vi "DataFlowExamples.vi"() -> ()   [LabVIEW 2020]
doc: "This VI have four examples of data flow using with good and bad habbits. Comments in polish language."
panel:
  out "Obecny czas 2":timestamp
  in  "Liczba 6":dbl
  in  "Liczba 5":dbl
  out "Wynik 3":dbl
  out "Obecny czas 1":timestamp
  out "Wynik 4":dbl
  in  "Liczba 7":dbl
  in  "Liczba 8":dbl
  in  "Liczba 3":dbl
  in  "Liczba 4":dbl
  out "Wynik 2":dbl
  out "Wynik 1":dbl
  in  "Liczba 2":dbl
  in  "Liczba 1":dbl
  # "Przykład 1"
  # "Przykład 2"
  # "Przykład 3"
  # "Przykład 4"
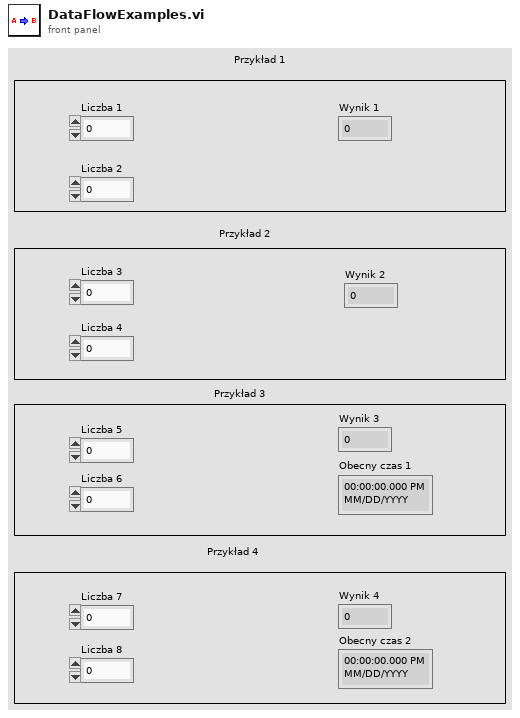
[diagram p1: front panel]
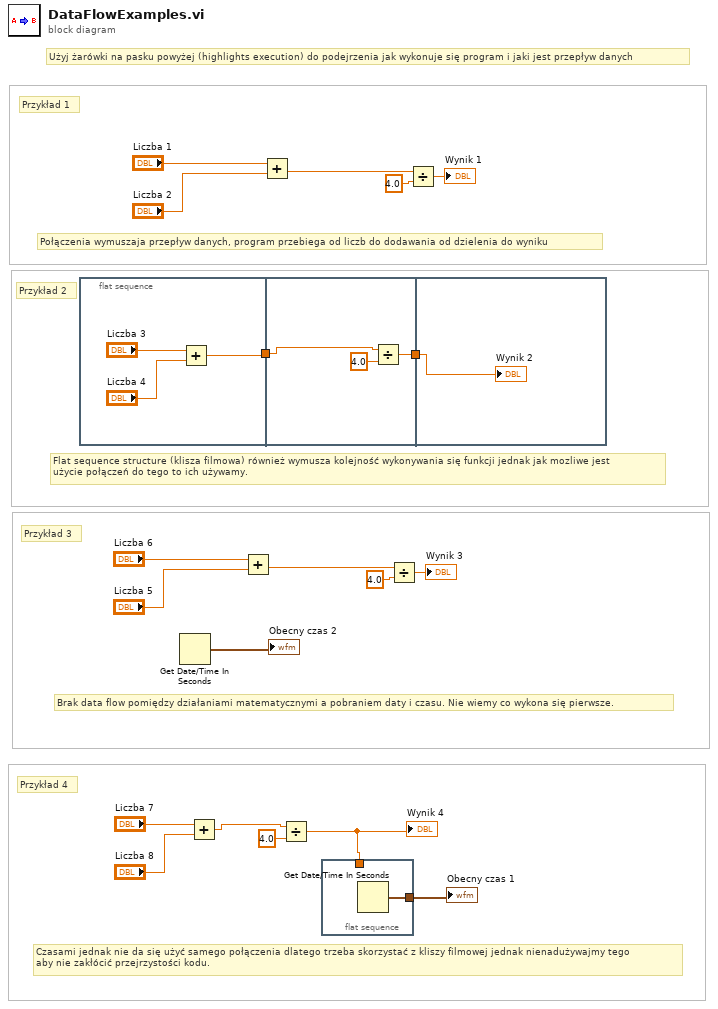
[diagram p0: block diagram]
diagram:
  # "Przykład 4"
  # "Przykład 3"
  # "Brak data flow pomiędzy działaniami matematycznymi a pobraniem daty i czasu. Nie wiemy co wykona się pierwsze."
  # "Przykład 2"
  # "Przykład 1"
  # "Czasami jednak nie da się użyć samego połączenia dlatego trzeba skorzystać z kliszy filmowej jednak nienadużywajmy tego\naby nie zakłócić przejrzystości kodu."
  # "Flat sequence structure (klisza filmowa) również wymusza kolejność wykonywania się funkcji jednak jak mozliwe jest\nużycie połączeń do tego to ich używamy."
  # "Użyj żarówki na pasku powyżej (highlights execution) do podejrzenia jak wykonuje się program i jaki jest przepływ danych"
  # "Połączenia wymuszaja przepływ danych, program przebiega od liczb do dodawania od dzielenia do wyniku"
  n1 = flat-sequence {
    tunnel: [w20] -> w13
    tunnel: [w24] -> w14
    tunnel: w13 -> [w23]
    tunnel: w14 -> [w26]
    frame #0 {
      n2 = Add(x="Liczba 3", y="Liczba 4") -> (x+y=w20:dbl)
    }
    frame #1 {
      n3 = Divide(x=w23, y=4.0) -> (x/y=w24:dbl)
    }
    frame #2 {
      "Wynik 2" <- w26
    }
  }
  n4 = Get Date/Time In Seconds() -> (seconds since 1Jan1904=→"Obecny czas 2":timestamp)
  n5 = Add(x="Liczba 7", y="Liczba 8") -> (x+y=w9:dbl)
  n6 = Add(x="Liczba 6", y="Liczba 5") -> (x+y=w4:dbl)
  n7 = Add(x="Liczba 1", y="Liczba 2") -> (x+y=w17:dbl)
  n8 = Divide(x=w9, y=4.0) -> (x/y=w8:dbl)
  "Wynik 4" <- w8
  n9 = flat-sequence {
    tunnel: w8 -> [_]
    tunnel: [w27] -> w7
    frame #0 {
      n10 = Get Date/Time In Seconds() -> (seconds since 1Jan1904=w27:timestamp)
    }
  }
  n11 = Divide(x=w4, y=4.0) -> (x/y=→"Wynik 3":dbl)
  n12 = Divide(x=w17, y=4.0) -> (x/y=→"Wynik 1":dbl)
  "Obecny czas 1" <- w7
